vi "String Indicator.vi"(10 "String Indicator":string, 11 "String Indicator in":refnum<class "String Indicator.lvclass">) -> (0 "error out":errorcluster)   [LabVIEW 2021, in "String Indicator Msg.lvlib" / "String Indicator.lvclass"]
uses:
  String Indicator.lvclass
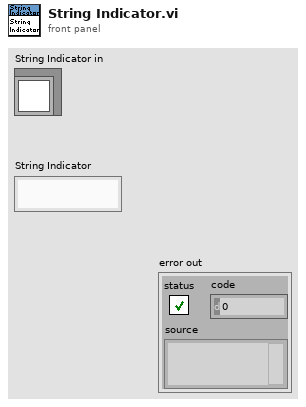
[diagram p1: front panel]
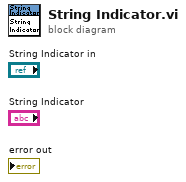
[diagram p0: block diagram]
diagram:
